vi "SEND SUBACK.vi"(8 "error in (no error)":errorcluster, 9 "Granted QoS Levels":T1(array[ring]), 10 "Message ID":u16=10 format="%x", 11 "connection ID":refnum<k5>) -> (0 "error out":errorcluster, 3 "connection ID out":refnum<k5>)   [LabVIEW 2025, in "DAQIO MQTT.lvlib"]
uses:
  DAQIO MQTT.lvlib
  Controls/MessageType.ctl
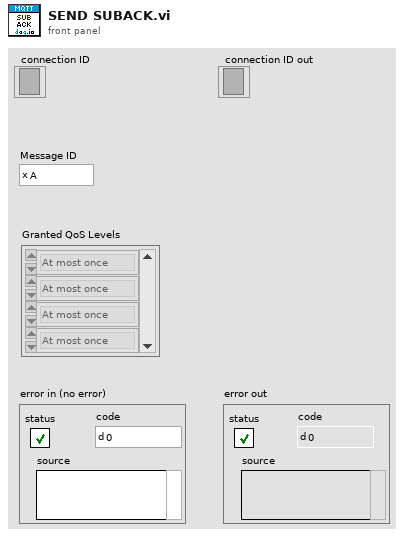
[diagram p1: front panel]
types:
  T1 = enum8{"At most once", "At least once", "Exactly once", "Reserved"}[]
  T2 = enum8{"At most once", "At least once", "Exactly once", "Reserved"}
  T3 = typedef "DAQIO MQTT.lvlib/MessageType.ctl" = enum32{"Reserved", "CONNECT", "CONNACK", "PUBLISH", "PUBACK", "PUBREC", "PUBREL", "PUBCOMP", "SUBSCRIBE", "SUBACK", "UNSUBSCRIBE", "UNSUBACK", "PINGREQ", "PINGRESP", "DISCONNECT", "Reserved2"}
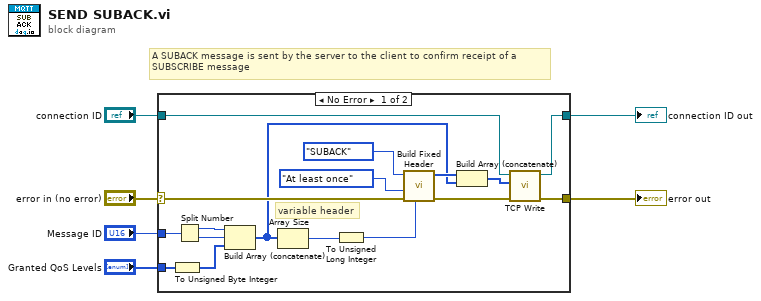
[diagram p0: block diagram]
diagram:
  # "A SUBACK message is sent by the server to the client to confirm receipt of a\nSUBSCRIBE message"
  n1 = case shown="No Error" "error in (no error)" {
    selector: "error in (no error)" -> [w18 w25]
    tunnel: [w13 w25] -> w5
    tunnel: "Granted QoS Levels" -> [w10 _]
    tunnel: "Message ID" -> [w9 _]
    tunnel: "connection ID" -> [w8 w24]
    tunnel: [w7 w24] -> w1
    frame No Error {
      # "variable header"
      n2 = To Unsigned Byte Integer(number=w10) -> (unsigned 8bit integer=w14:u8[])
      n3 = Split Number(x=w9) -> (hi(x)=w21:u8, lo(x)=w20:u8)
      n4 = Build Array (concatenate)(w21, w20, w14) -> (w17:u8[])
      n5 = Array Size(array=w17) -> (size(s)=w16:i32)
      n6 = To Unsigned Long Integer(number=w16) -> (unsigned 32bit integer=w15:u32)
      n7 = call "Build Fixed Header.vi"("Remaining Length"=w15, "error in (no error)"=w18, "QoS"=T2."At least once", "MessageType"=MessageType."SUBACK") -> ("error out"=w12:errorcluster, "Fixed Header"=w22:u8[])  [unwired: 6 in]
      n8 = Build Array (concatenate)(w22, w17) -> (w11:u8[])
      n9 = call "TCP Write.vi"("error in (no error)"=w12, "data in"=w11, "connection ID"=w8) -> ("error out"=w13:errorcluster, "connection ID out"=w7:refnum<k5>)  [unwired: 6 in, 1 out]
    }
    frame Error {
    }
  }
  "error out" <- w5
  "connection ID out" <- w1
